vi "Arrange GU Dialog.vi"(6 "Enabled Site":i32[](array[numeric])=[0, 2], 7 "CAL Config File Path":path=path "C:/Users/Public/Documents/National Instruments/Golden Units Calibration Tool/Calibration Config/Golden Units Calibration.csv", 8 "error in":errorcluster, 9 "Cur Cal Type":T2=enum."Check", 10 "All Available GU":i32[](array[numeric])=[1, 2, 3], 11 "Config File Data":T1(array[cluster])=[{"Section Name"="General", "Section Data"=[["Match_SeqFile", "Golden Units Calibration.seq"], ["CorrOffsetFilePath", "C:\\Users\\Public\\Documents\\National Instruments\\TestStand 2019 (64-bit)\\Examples\\Golden Units Calibration Tool\\Supporting Materials\\Golden Units\\Offset.txt"]]}, {"Section Name"="PluginCfg", "Section Data"=[["GUCalibration.lvlib", "Enabled:TRUE;Trigger:TRUE;Option:TRUE;Limit:TRUE;Offset:TRUE;Report:TRUE"]]}, {"Section Name"="PluginSpecific", "Section Data"=[["CorrOffsetFilePath", "C:\\Users\\Public\\Documents\\National Instruments\\TestStand 2019 (64-bit)\\Examples\\Golden Units Calibration Tool\\Supporting Materials\\Golden Units\\Offset.txt"], ["GUBenchFilePath", "C:\\Users\\Public\\Documents\\National Instruments\\TestStand 2019 (64-bit)\\Examples\\Golden Units Calibration Tool\\Supporting Materials\\Golden Units\\GU_Bench.csv"], ["IsCalibration", "FALSE"]]}, {"Section Name"="CalCfg", "Section Data"=[["Index", "TestName", "TestNumber", "Units", "LowLimit", "HighLimit", "GU_1"], ["1", "TXP - Average Mean Power", "1001", "dBm", "-13", "-11", "0"], ["2", "TXP - Peak to Average Ratio", "1002", "dB", "9", "11", "0"], ["3", "TXP - Maximum Power", "1003", "dBm", "-3", "-1", "0"], ["4", "TXP - Minimum Power", "1004", "dBm", "0", "0", "0"], ["5", "AMPM - Mean RMS EVM", "2001", "%", "0.1", "0.3", "0"], ["6", "AMPM - Mean Linear Gain", "2002", "dB", "-4", "-2", "0"]]}]) -> (0 "error out":errorcluster, 1 "Msg":string, 3 "Config File.Data":T1(array[cluster])=[{"Section Name"="General", "Section Data"=[["Match_SeqFile", "Golden Units Calibration.seq"], ["CorrOffsetFilePath", "C:\\Users\\Public\\Documents\\National Instruments\\TestStand 2019 (64-bit)\\Examples\\Golden Units Calibration Tool\\Supporting Materials\\Golden Units\\Offset.txt"]]}, {"Section Name"="PluginCfg", "Section Data"=[["GUCalibration.lvlib", "Enabled:TRUE;Trigger:TRUE;Option:TRUE;Limit:TRUE;Offset:TRUE;Report:TRUE"]]}, {"Section Name"="PluginSpecific", "Section Data"=[["CorrOffsetFilePath", "C:\\Users\\Public\\Documents\\National Instruments\\TestStand 2019 (64-bit)\\Examples\\Golden Units Calibration Tool\\Supporting Materials\\Golden Units\\Offset.txt"], ["GUBenchFilePath", "C:\\Users\\Public\\Documents\\National Instruments\\TestStand 2019 (64-bit)\\Examples\\Golden Units Calibration Tool\\Supporting Materials\\Golden Units\\GU_Bench.csv"], ["IsCalibration", "FALSE"]]}, {"Section Name"="CalCfg", "Section Data"=[["Index", "TestName", "TestNumber", "Units", "LowLimit", "HighLimit", "GU_1"], ["1", "TXP - Average Mean Power", "1001", "dBm", "-13", "-11", "0"], ["2", "TXP - Peak to Average Ratio", "1002", "dB", "9", "11", "0"], ["3", "TXP - Maximum Power", "1003", "dBm", "-3", "-1", "0"], ["4", "TXP - Minimum Power", "1004", "dBm", "0", "0", "0"], ["5", "AMPM - Mean RMS EVM", "2001", "%", "0.1", "0.3", "0"], ["6", "AMPM - Mean Linear Gain", "2002", "dB", "-4", "-2", "0"]]}, {"Section Name"="Backup", "Section Data"=[["CorrOffsetFilePath", "C:\\Users\\Public\\Documents\\National Instruments\\TestStand 2019 (64-bit)\\Examples\\Golden Units Calibration Tool\\Supporting Materials\\Golden Units\\Offset.txt"], ["GUBenchFilePath", "C:\\Users\\Public\\Documents\\National Instruments\\TestStand 2019 (64-bit)\\Examples\\Golden Units Calibration Tool\\Supporting Materials\\Golden Units\\GU_Bench.csv"], ["IsCalibration", "FALSE"]]}])   [LabVIEW 2020, in "GUCalibration2.lvlib"]
uses:
  GUCalibration2.lvlib
  Controls/CalibrationOrCheck.ctl
  Controls/GU Arrange UI Ref.ctl
  Controls/Config Data Type.ctl
  Controls/GU Arrange Check Rule.ctl
panel:
  in  "Tab":enum32{"GU Selection", "GU Distribution"}(tab)
  in  "Abort":bool
  in  "Next":bool
  out "Selected GU List":i32(listbox)
  in  "Availabe GU List":i32(listbox)
  in  "Select All":bool
  in  "Select None":bool
  in  "GU Arrange List":i32(listbox)
  in  "Auto Arrange":bool
  in  "OK":bool
  in  "Back":bool
  in  "Loop Count per GU":i32=1 min=1 step=1
  in  "Min Num of Pass GUs per Site":i32=1 min=1 step=1
  # "Select GUs"
  # "GU Arrangements"
  # "Arrangement"
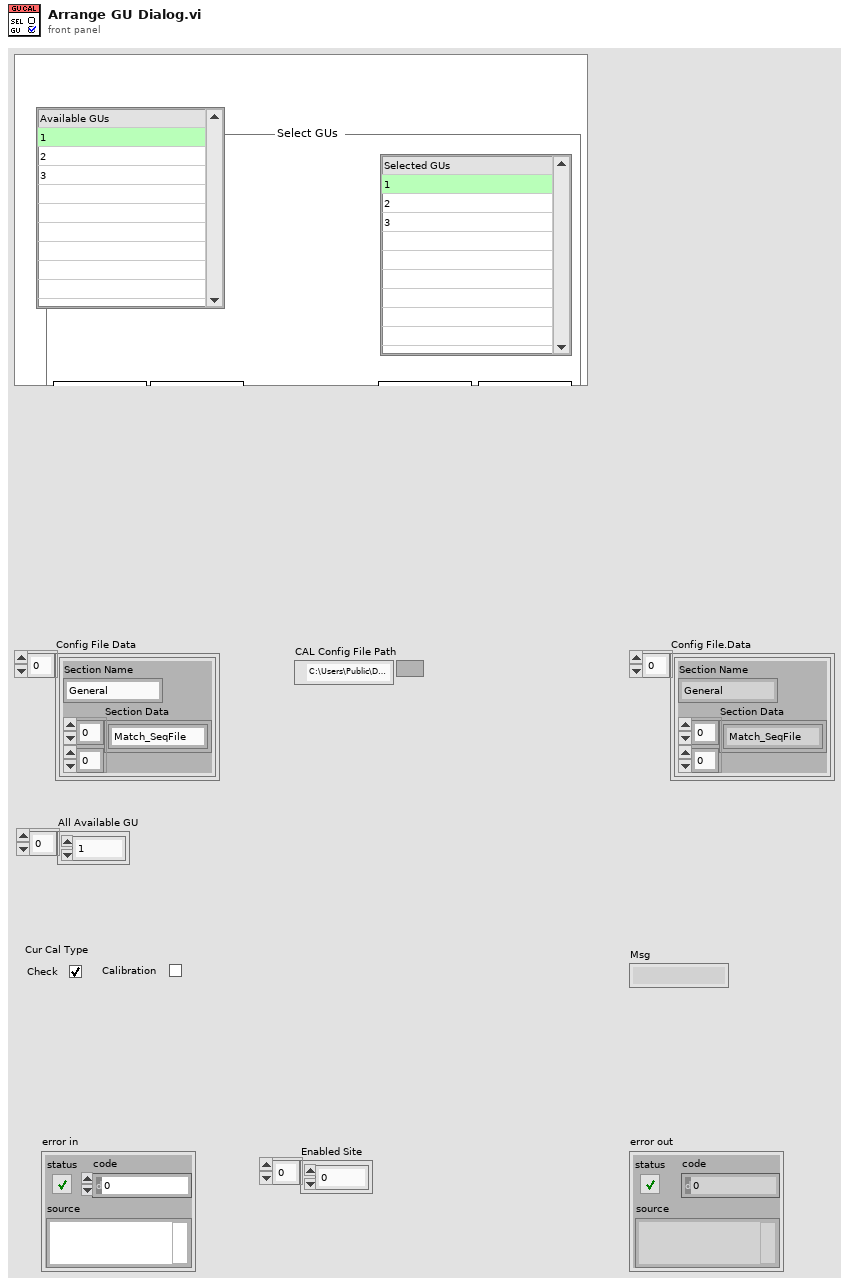
[diagram p1: front panel]
types:
  T1 = cluster{"Section Name":string, "Section Data":string[][]}[]
  T2 = typedef "GUCalibration2.lvlib/CalibrationOrCheck.ctl" = enum32{"Calibration", "Check"}
  T3 = typedef "GUCalibration2.lvlib/GU Arrange UI Ref.ctl" = cluster{"Availabe GU List":refnum<vi>, "Selected GU List":refnum<vi>, "Tab":refnum<vi>, "GU Arrange List":refnum<vi>, "Loop Count Per Batch":refnum<vi>, "This VI":refnum<vi>, "Min Num of Pass Batch":refnum<vi>}
  T4 = typedef "GUCalibration2.lvlib/Config Data Type.ctl" = cluster{"Cal Type":i32, "Curr Batch Index":i32, "Loop Count Per GU":i32, "Min Num of Pass GUs Per Site":i32, "Is Calibration":bool, "Batch Iteration Done":bool, "Cal Abort":bool, "Update Offset":bool, "Cal Check Pass":bool, "Cal End":bool, "Enabled Site":i32[], "GU Selected":i32[], "All Available GU":i32[], "GU Arrange":i32[][], "Batch Test Count":i32[][], "Batch Test Result":string[][], "Curr Batch":i32[], "Curr Batch Test Count":i32[], "Curr Batch Target Count":i32[], "Curr Batch Test Result":string[]}
  T5 = typedef "GUCalibration2.lvlib/GU Arrange Check Rule.ctl" = enum16{"Invalid GU Number", "GU Number Conflict"}
  T6 = cluster{"Error In":errorcluster, "Config File":cluster{"Path":path, "Data":cluster{"Section Name":string, "Section Data":string[][]}[], "Data Backup":cluster{"Section Name":string, "Section Data":string[][]}[]}, "Ctrl Ref":T3, "Latest Cal Data":T4, "Curr Cal Cfg":T4, "Items Pre Edit":string[][], "Error Cell":cluster{"Cell Pos":cluster{"Row":i32, "Column":i32}[], "Error Msg":T5}[], "Exit":bool, "msg":string}
  T7 = typedef "LVPoint32TypeDef.ctl" = cluster{"Horizontal":i32, "Vertical":i32}
  T8 = typedef "LVRowAndColumnTypeDef.ctl" = cluster{"Row":i32, "Column":i32}
  T9 = cluster{"Cell Pos":cluster{"Row":i32, "Column":i32}[], "Error Msg":T5}[]
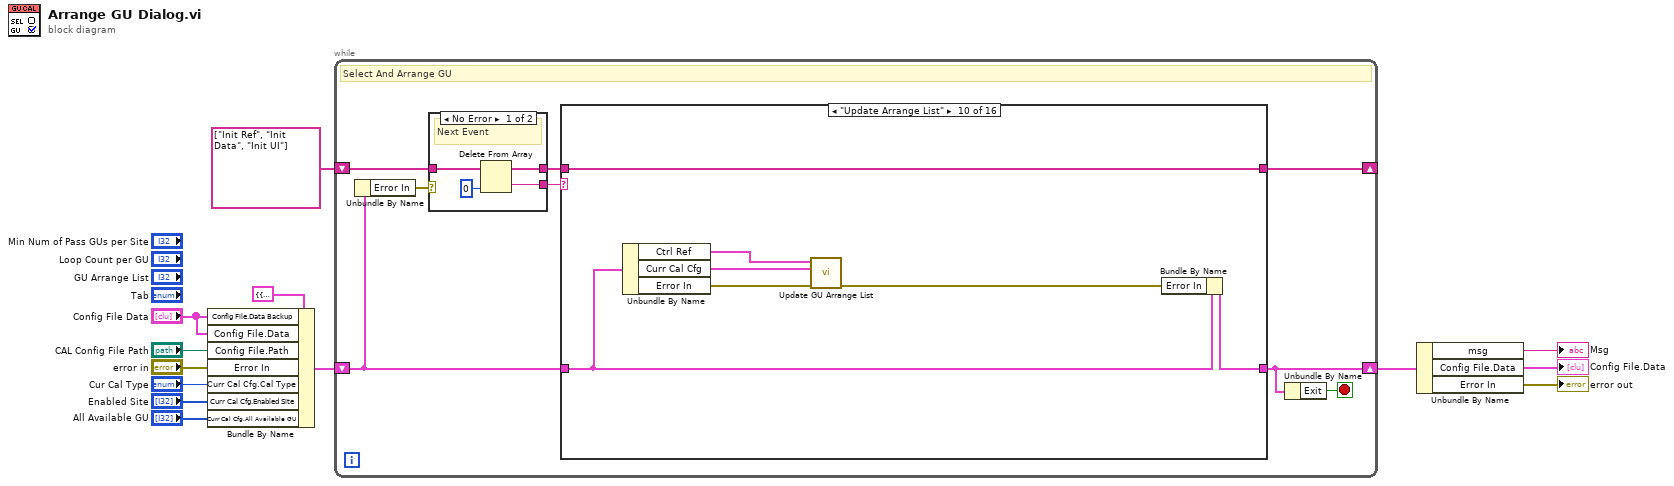
[diagram p0: block diagram]
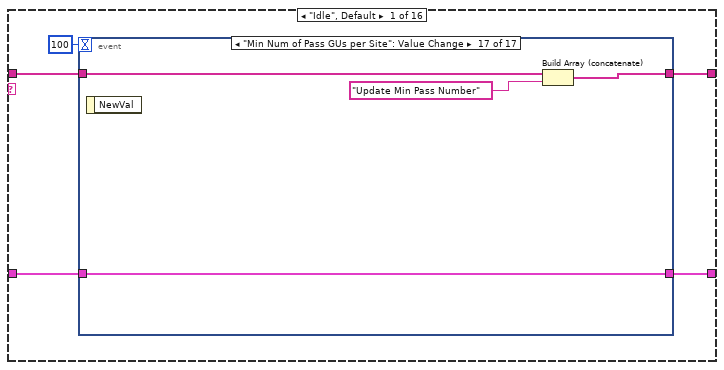
[diagram p2: hidden frame]
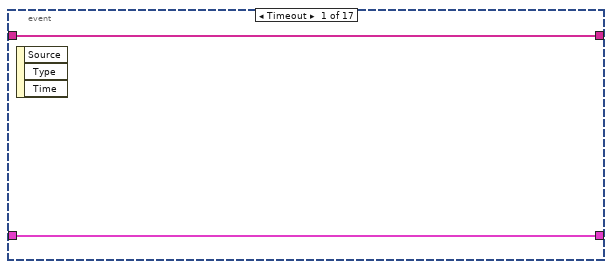
[diagram p3: hidden frame]
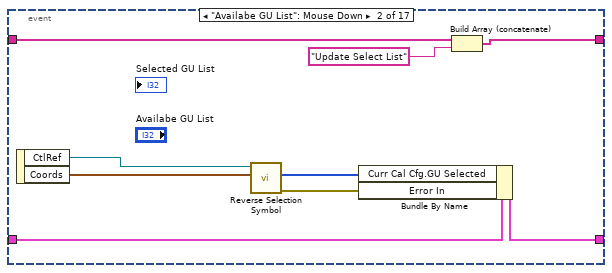
[diagram p4: hidden frame]
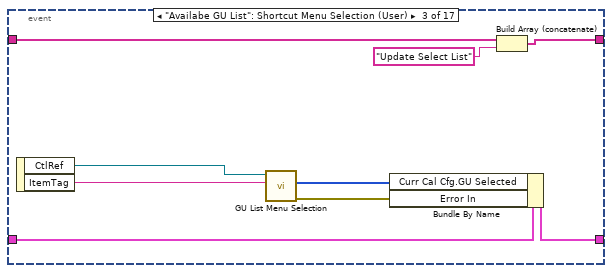
[diagram p5: hidden frame]
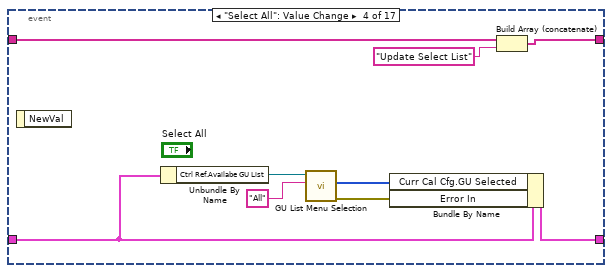
[diagram p6: hidden frame]
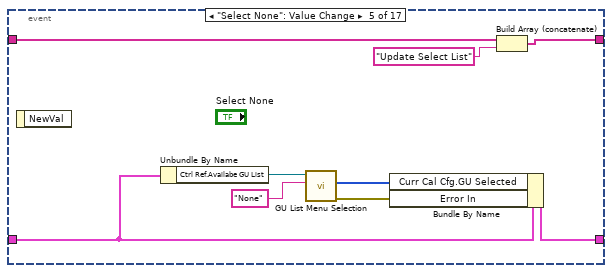
[diagram p7: hidden frame]
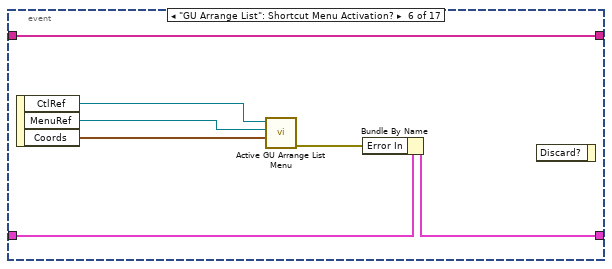
[diagram p8: hidden frame]
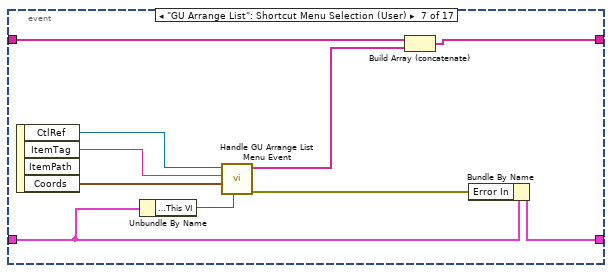
[diagram p9: hidden frame]
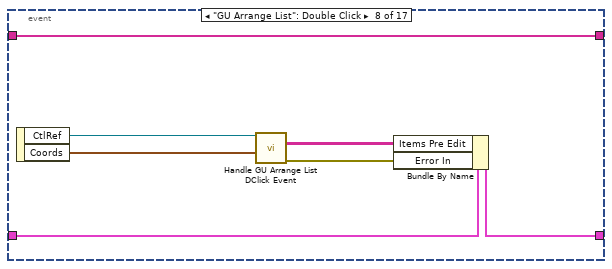
[diagram p10: hidden frame]
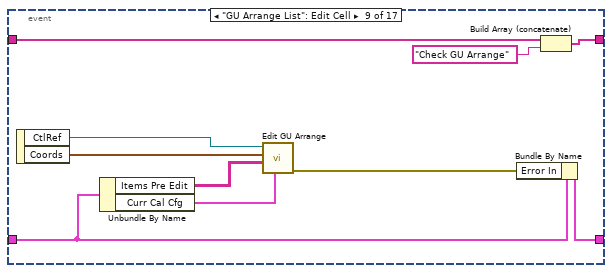
[diagram p11: hidden frame]
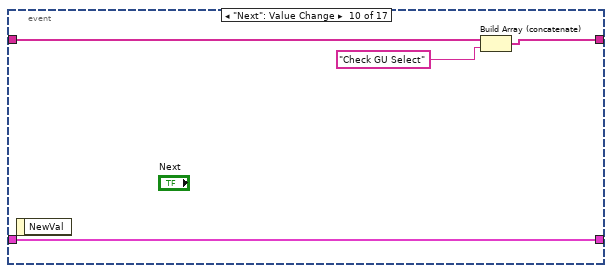
[diagram p12: hidden frame]
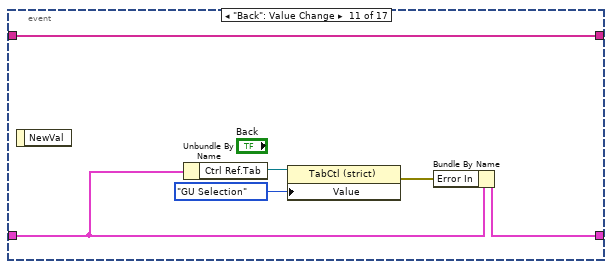
[diagram p13: hidden frame]
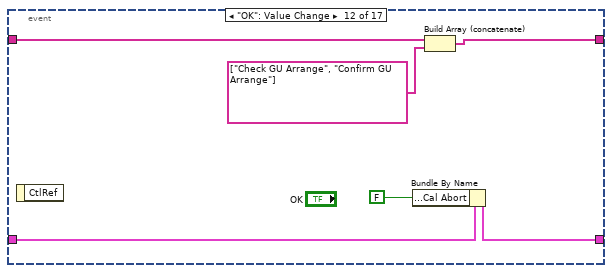
[diagram p14: hidden frame]
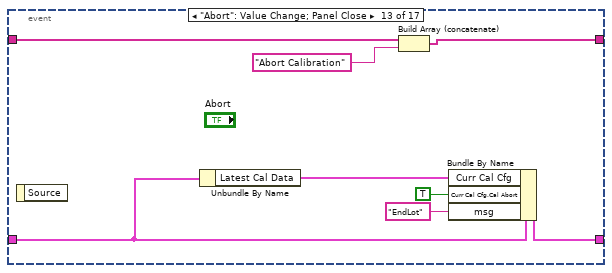
[diagram p15: hidden frame]
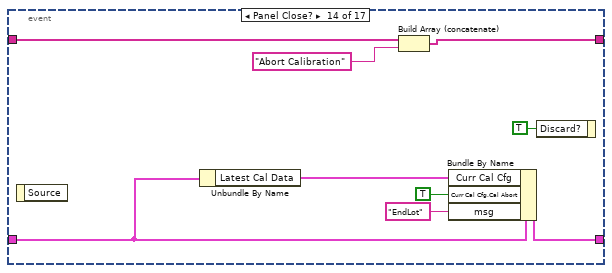
[diagram p16: hidden frame]
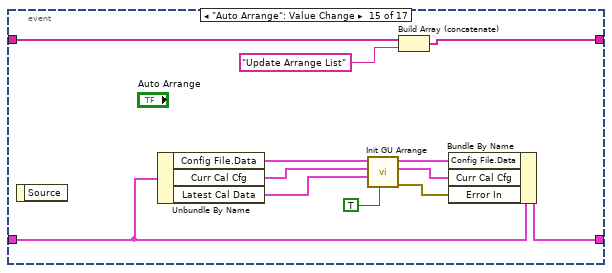
[diagram p17: hidden frame]
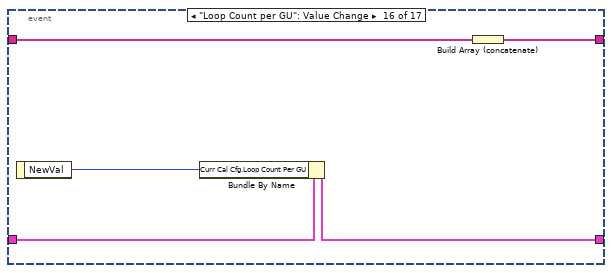
[diagram p18: hidden frame]
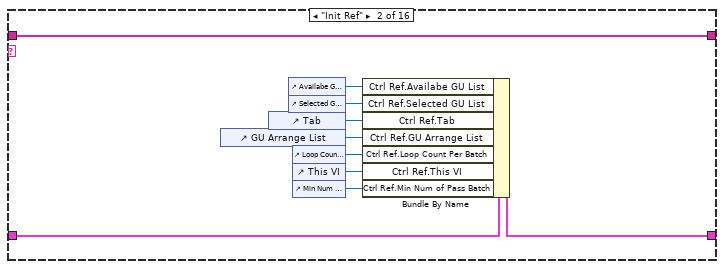
[diagram p19: hidden frame]
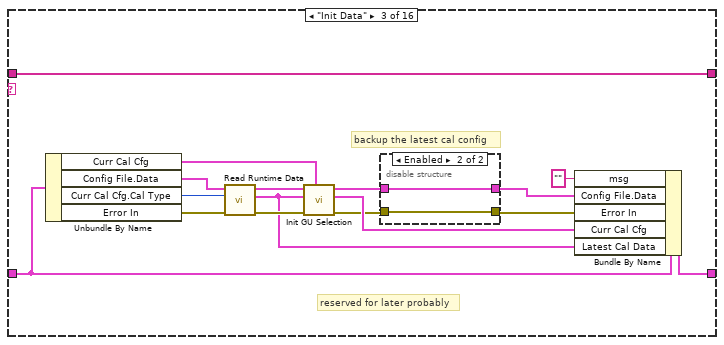
[diagram p20: hidden frame]
diagram:
  n1 = Bundle By Name(cluster=T6 {"Error In"={"status"=FALSE, "code"=0, "source"=""}, "Config File"={"Path"=path "", "Data"=[], "Data Backup"=[]}, "Ctrl Ref"={"Availabe GU List"=refnum, "Selected GU List"=refnum, "Tab"=refnum, "GU Arrange List"=refnum, "Loop Count Per Batch"=refnum, "This VI"=refnum, "Min Num of Pass Batch"=refnum}, "Latest Cal Data"={"Cal Type"=0, "Curr Batch Index"=0, "Loop Count Per GU"=0, "Min Num of Pass GUs Per Site"=0, "Is Calibration"=FALSE, "Batch Iteration Done"=FALSE, "Cal Abort"=FALSE, "Update Offset"=FALSE, "Cal Check Pass"=FALSE, "Cal End"=FALSE, "Enabled Site"=[], "GU Selected"=[], "All Available GU"=[], "GU Arrange"=[], "Batch Test Count"=[], "Batch Test Result"=[], "Curr Batch"=[], "Curr Batch Test Count"=[], "Curr Batch Target Count"=[], "Curr Batch Test Result"=[]}, "Curr Cal Cfg"={"Cal Type"=0, "Curr Batch Index"=0, "Loop Count Per GU"=0, "Min Num of Pass GUs Per Site"=0, "Is Calibration"=FALSE, "Batch Iteration Done"=FALSE, "Cal Abort"=FALSE, "Update Offset"=FALSE, "Cal Check Pass"=FALSE, "Cal End"=FALSE, "Enabled Site"=[], "GU Selected"=[], "All Available GU"=[], "GU Arrange"=[], "Batch Test Count"=[], "Batch Test Result"=[], "Curr Batch"=[], "Curr Batch Test Count"=[], "Curr Batch Target Count"=[], "Curr Batch Test Result"=[]}, "Items Pre Edit"=[], "Error Cell"=[], "Exit"=FALSE, "msg"=""} ("Temp Var"), "Config File.Data Backup"="Config File Data", "Config File.Data"="Config File Data", "Config File.Path"="CAL Config File Path", "Error In"="error in", "Curr Cal Cfg.Cal Type"="Cur Cal Type", "Curr Cal Cfg.Enabled Site"="Enabled Site", "Curr Cal Cfg.All Available GU"="All Available GU") -> (w10:T6)
  n2 = while {
    shift-right: [w18] -> _
    shift-left: string[] ["Init Ref", "Init Data", "Init UI"] ("Array") -> [w21]
    shift-right: [w15] -> w9
    shift-left: w10 -> [w14]
    stop <- w16 stop-if-true
    # "Select And Arrange GU"
    n3 = Unbundle By Name(w14) -> ("Error In"=w20:errorcluster)
    n4 = case shown="No Error" w20 {
      tunnel: w21 -> [w310 w312]
      tunnel: [w308 w312] -> w19
      tunnel: [w307 "Error Handle" ("String")] -> w17
      frame No Error {
        # "Next Event"
        n5 = Delete From Array(array=w310, index=0) -> (deleted portion=w307:string, array with subset deleted=w308:string[])  [unwired: 1 in]
      }
      frame Error {
        # "Error Event"
      }
    }
    n6 = case shown="\"Update Arrange List\"" w17 {
      tunnel: [w25 w160 w176 w195 w203 w208 w213 w217 w218 w229 w240 w253 w265 w279 w295 w299] -> w15
      tunnel: w14 -> [w24 w161 w175 w194 w204 w209 w214 w217 w219 w230 w242 w251 w266 w280 w296 w300]
      tunnel: w19 -> [w23 w162 w178 w196 w205 w211 w215 w216 w224 w231 w243 w254 w272 w275 w293 w306]
      tunnel: [w22 w162 w178 w196 w205 w211 w215 w216 w224 w231 w243 w245 w263 w274 w292 w306] -> w18
      frame "Idle", Default {
        n7 = event shown="[16] \"Min Num of Pass GUs per Site\": Value Change" {
          selector: _ -> [_ _ _ _ _ _ _ _ _ _ _ _ _ _ _ _ _]
          dyn-events: _ -> [_ _ _ _ _ _ _ _ _ _ _ _ _ _ _ _ _]
          timeout: 100 -> [_ _ _ _ _ _ _ _ _ _ _ _ _ _ _ _ _]
          tunnel: [w28 w33 w43 w55 w64 w66 w78 w86 w93 w101 w104 w111 w122 w131 w143 w146 w149] -> w25
          tunnel: w24 -> [w28 w34 w46 w49 w58 w71 w73 w88 w98 w101 w107 w109 w117 w126 w140 w148 w149]
          tunnel: w23 -> [w27 w37 w39 w51 w60 w70 w76 w87 w91 w102 w108 w114 w119 w128 w142 w147 w152]
          tunnel: [w27 w30 w38 w50 w59 w70 w74 w87 w90 w100 w108 w113 w118 w127 w141 w144 w151] -> w22
          event Timeout {
            n8 = event-data() -> ()  [unwired: 1 in, 3 out]
          }
          event "Availabe GU List": Mouse Down {
            n9 = event-data() -> ("CtlRef"=w35:refnum<vi>, "Coords"=w36:T7)  [unwired: 1 in]
            n10 = call "Reverse Selection Symbol.vi"("Coords"=w36, "GU List Ref"=w35) -> ("error out"=w32:errorcluster, "Selected GU"=w31:i32[])  [unwired: 8 in]
            n11 = Bundle By Name(cluster=w34, "Curr Cal Cfg.GU Selected"=w31, "Error In"=w32) -> (w33:T6)
            n12 = Build Array (concatenate)(w37, "Update Select List" ("String")) -> (w30:string[])
          }
          event "Availabe GU List": Shortcut Menu Selection (User) {
            n13 = event-data() -> ("CtlRef"=w45:refnum<vi>, "ItemTag"=w44:string)  [unwired: 1 in]
            n14 = call "GU List Menu Selection.vi"("ItemTag"=w44, "CtlRef"=w45) -> ("error out"=w42:errorcluster, "Selected GU"=w41:i32[])  [unwired: 8 in]
            n15 = Bundle By Name(cluster=w46, "Curr Cal Cfg.GU Selected"=w41, "Error In"=w42) -> (w43:T6)
            n16 = Build Array (concatenate)(w39, "Update Select List" ("String")) -> (w38:string[])
          }
          event "Select All": Value Change {
            n17 = event-data() -> ()  [unwired: 1 in, 1 out]
            n18 = Unbundle By Name(w49) -> ("Ctrl Ref.Availabe GU List"=w48:refnum<vi>)
            n19 = call "GU List Menu Selection.vi"("ItemTag"="All", "CtlRef"=w48) -> ("error out"=w54:errorcluster, "Selected GU"=w53:i32[])  [unwired: 8 in]
            n20 = Bundle By Name(cluster=w49, "Curr Cal Cfg.GU Selected"=w53, "Error In"=w54) -> (w55:T6)
            n21 = Build Array (concatenate)(w51, "Update Select List" ("String")) -> (w50:string[])
          }
          event "Select None": Value Change {
            n22 = event-data() -> ()  [unwired: 1 in, 1 out]
            n23 = Unbundle By Name(w58) -> ("Ctrl Ref.Availabe GU List"=w57:refnum<vi>)
            n24 = call "GU List Menu Selection.vi"("ItemTag"="None", "CtlRef"=w57) -> ("error out"=w63:errorcluster, "Selected GU"=w62:i32[])  [unwired: 8 in]
            n25 = Bundle By Name(cluster=w58, "Curr Cal Cfg.GU Selected"=w62, "Error In"=w63) -> (w64:T6)
            n26 = Build Array (concatenate)(w60, "Update Select List" ("String")) -> (w59:string[])
          }
          event "GU Arrange List": Shortcut Menu Activation? {
            n27 = event-data() -> ("CtlRef"=w69:refnum<vi>, "MenuRef"=w68:refnum<k9>, "Coords"=w67:T7)  [unwired: 1 in]
            n28 = call "Active GU Arrange List Menu.vi"("Point"=w67, "MenuRef"=w68, "CtlRef"=w69) -> ("error out"=w65:errorcluster)  [unwired: 8 in]
            n29 = Bundle By Name(cluster=w71, "Error In"=w65) -> (w66:T6)
            n30 = event-data() -> ()  [unwired: 2 in, 1 out]
          }
          event "GU Arrange List": Shortcut Menu Selection (User) {
            n31 = event-data() -> ("CtlRef"=w79:refnum<vi>, "ItemTag"=w80:string, "Coords"=w81:T7)  [unwired: 1 in, 1 out]
            n32 = Unbundle By Name(w73) -> ("Ctrl Ref.This VI"=w72:refnum<vi>)
            n33 = call "Handle GU Arrange List Menu Event.vi"("Top VI"=w72, "Coords"=w81, "ItemTag"=w80, "CtlRef"=w79) -> ("error out"=w77:errorcluster, "Next Case"=w75:string[])  [unwired: 6 in]
            n34 = Build Array (concatenate)(w76, w75) -> (w74:string[])
            n35 = Bundle By Name(cluster=w73, "Error In"=w77) -> (w78:T6)
          }
          event "GU Arrange List": Double Click {
            n36 = event-data() -> ("CtlRef"=w85:refnum<vi>, "Coords"=w84:T7)  [unwired: 1 in]
            n37 = call "Handle GU Arrange List DClick Event.vi"("Coords"=w84, "CtlRef"=w85) -> ("error out"=w83:errorcluster, "Item Names"=w82:string[][])  [unwired: 8 in]
            n38 = Bundle By Name(cluster=w88, "Items Pre Edit"=w82, "Error In"=w83) -> (w86:T6)
          }
          event "GU Arrange List": Edit Cell {
            n39 = event-data() -> ("CtlRef"=w95:refnum<vi>, "Coords"=w96:T8)  [unwired: 1 in]
            n40 = Unbundle By Name(w98) -> ("Items Pre Edit"=w97:string[][], "Curr Cal Cfg"=w94:T4)
            n41 = call "Edit GU Arrange.vi"("Curr Cal Cfg In"=w94, "Items Pre Edit"=w97, "Coords"=w96, "CtlRef"=w95) -> ("error out"=w92:errorcluster)  [unwired: 7 in]
            n42 = Bundle By Name(cluster=w98, "Error In"=w92) -> (w93:T6)
            n43 = Build Array (concatenate)(w91, "Check GU Arrange" ("String")) -> (w90:string[])
          }
          event "Next": Value Change {
            n44 = event-data() -> ()  [unwired: 1 in, 1 out]
            n45 = Build Array (concatenate)(w102, "Check GU Select" ("String")) -> (w100:string[])
          }
          event "Back": Value Change {
            n46 = event-data() -> ()  [unwired: 1 in, 1 out]
            n47 = Unbundle By Name(w107) -> ("Ctrl Ref.Tab"=w106:refnum<vi>)
            n48 = property class="TabCtl (strict)"(reference=w106, "Value"=enum32{"GU Selection", "GU Distribution"}."GU Selection") -> (error out=w103:errorcluster)  [unwired: 1 in, 1 out]
            n49 = Bundle By Name(cluster=w107, "Error In"=w103) -> (w104:T6)
          }
          event "OK": Value Change {
            n50 = event-data() -> ()  [unwired: 1 in, 1 out]
            n51 = Bundle By Name(cluster=w109, "Curr Cal Cfg.Cal Abort"=FALSE ("Cal Abort")) -> (w111:T6)
            n52 = Build Array (concatenate)(w114, string[] ["Check GU Arrange", "Confirm GU Arrange"] ("Array")) -> (w113:string[])
          }
          event "Abort": Value Change; Panel Close {
            n53 = event-data() -> ()  [unwired: 1 in, 1 out]
            n54 = Unbundle By Name(w117) -> ("Latest Cal Data"=w116:T4)
            n55 = Build Array (concatenate)(w119, "Abort Calibration" ("msg")) -> (w118:string[])
            n56 = Bundle By Name(cluster=w117, "Curr Cal Cfg"=w116, "Curr Cal Cfg.Cal Abort"=TRUE, "msg"="EndLot") -> (w122:T6)
          }
          event Panel Close? {
            n57 = event-data() -> ()  [unwired: 1 in, 1 out]
            n58 = Unbundle By Name(w126) -> ("Latest Cal Data"=w125:T4)
            n59 = Build Array (concatenate)(w128, "Abort Calibration" ("msg")) -> (w127:string[])
            n60 = Bundle By Name(cluster=w126, "Curr Cal Cfg"=w125, "Curr Cal Cfg.Cal Abort"=TRUE, "msg"="EndLot") -> (w131:T6)
            n61 = event-data("Discard?"=TRUE) -> ()  [unwired: 1 in, 1 out]
          }
          event "Auto Arrange": Value Change {
            n62 = event-data() -> ()  [unwired: 1 in, 1 out]
            n63 = Unbundle By Name(w140) -> ("Config File.Data"=w138:T1, "Curr Cal Cfg"=w137:T4, "Latest Cal Data"=w136:T4)
            n64 = call "Init GU Arrange.vi"("Force Auto(False)"=TRUE, "Latest Cal Cfg"=w136, "Curr Cal Cfg In"=w137, "Config Data"=w138) -> ("error out"=w133:errorcluster, "Curr Cal Cfg Out"=w134:T4, "Config Data Out"=w135:T1)  [unwired: 5 in]
            n65 = Build Array (concatenate)(w142, "Update Arrange List" ("msg")) -> (w141:string[])
            n66 = Bundle By Name(cluster=w140, "Config File.Data"=w135, "Curr Cal Cfg"=w134, "Error In"=w133) -> (w143:T6)
          }
          event "Loop Count per GU": Value Change {
            n67 = event-data() -> ("NewVal"=w145:i32)  [unwired: 1 in]
            n68 = Bundle By Name(cluster=w148, "Curr Cal Cfg.Loop Count Per GU"=w145) -> (w146:T6)
            n69 = Build Array (concatenate)(w147) -> (w144:string[])
          }
          event "Min Num of Pass GUs per Site": Value Change {
            n70 = event-data() -> ()  [unwired: 1 in, 1 out]
            n71 = Build Array (concatenate)(w152, "Update Min Pass Number" ("String")) -> (w151:string[])
          }
        }
      }
      frame "Init Ref" {
        n72 = control-ref of="GU Arrange List"() -> (w156:refnum<vi>)
        n73 = control-ref of="Tab"() -> (w157:refnum<vi>)
        n74 = control-ref of="Availabe GU List"() -> (w159:refnum<vi>)
        n75 = control-ref of="Selected GU List"() -> (w158:refnum<vi>)
        n76 = control-ref of="Loop Count per GU"() -> (w155:refnum<vi>)
        n77 = control-ref of="This VI"() -> (w154:refnum<vi>)
        n78 = control-ref of="Min Num of Pass GUs per Site"() -> (w153:refnum<vi>)
        n79 = Bundle By Name(cluster=w161, "Ctrl Ref.Availabe GU List"=w159, "Ctrl Ref.Selected GU List"=w158, "Ctrl Ref.Tab"=w157, "Ctrl Ref.GU Arrange List"=w156, "Ctrl Ref.Loop Count Per Batch"=w155, "Ctrl Ref.This VI"=w154, "Ctrl Ref.Min Num of Pass Batch"=w153) -> (w160:T6)
      }
      frame "Init Data" {
        # "reserved for later probably"
        # "backup the latest cal config"
        n80 = Unbundle By Name(w175) -> ("Curr Cal Cfg"=w168:T4, "Config File.Data"=w177:T1, "Curr Cal Cfg.Cal Type"=w163:i32, "Error In"=w167:errorcluster)
        n81 = call "Read Runtime Data.vi"("error in"=w167, "Curr Cal Type"=w163, "Config File Data In"=w177) -> ("error out"=w174:errorcluster, "Runtime Data Out"=w173:T4, "Config Data Out"=w172:T1)  [unwired: 6 in]
        n82 = call "Init GU Selection.vi"("Curr Cal Cfg In"=w168, "error in"=w174, "Latest Cal Cfg"=w173, "Config Data"=w172) -> ("error out"=w166:errorcluster, "Curr Cal Cfg Out"=w169:T4, "Config Data Out"=w165:T1)  [unwired: 5 in]
        n83 = disable-structure shown="Enabled" {
          disable-tunnel: [w184 w185] -> w171
          disable-tunnel: [w183 w186] -> w170
          disable-tunnel: w166 -> [w182 w185]
          disable-tunnel: w165 -> [w181 w186]
          frame Disabled {
            n84 = call "Remove Backup Config.vi"("error in"=w182, "Config File Data In"=w181) -> ("error out"=w179:errorcluster, "Config Data Out"=w180:T1)  [unwired: 8 in]
            n85 = call "Backup Latest Cal Config.vi"("error in"=w179, "Config File Data In"=w180) -> ("error out"=w184:errorcluster, "Config Data Out"=w183:T1)  [unwired: 8 in]
          }
          frame Enabled {
          }
        }
        n86 = Bundle By Name(cluster=w175, "msg"="", "Config File.Data"=w170, "Error In"=w171, "Curr Cal Cfg"=w169, "Latest Cal Data"=w173) -> (w176:T6)
      }
      frame "Init GU Arrange" {
        n87 = Unbundle By Name(w194) -> ("Config File.Data"=w192:T1, "Curr Cal Cfg"=w191:T4, "Latest Cal Data"=w190:T4, "Error In"=w193:errorcluster)
        n88 = call "Init GU Arrange.vi"("error in"=w193, "Latest Cal Cfg"=w190, "Curr Cal Cfg In"=w191, "Config Data"=w192) -> ("error out"=w189:errorcluster, "Curr Cal Cfg Out"=w187:T4, "Config Data Out"=w188:T1)  [unwired: 5 in]
        n89 = Bundle By Name(cluster=w194, "Config File.Data"=w188, "Curr Cal Cfg"=w187, "Error In"=w189) -> (w195:T6)
      }
      frame "Init UI" {
        n90 = Unbundle By Name(w204) -> ("Curr Cal Cfg"=w201:T4, "Ctrl Ref"=w199:T3, "Latest Cal Data.Loop Count Per GU"=w197:i32, "Error In"=w198:errorcluster)
        n91 = call "Init Front Panel Ctrls.vi"("error in"=w198, "Latest Loop Count"=w197, "Ctrl Ref"=w199) -> ("error out"=w200:errorcluster)  [unwired: 8 in]
        n92 = call "Update GU Selection List.vi"("error in"=w200, "Curr Cal Cfg"=w201, "Ctrl Ref"=w199) -> ("error out"=w202:errorcluster)  [unwired: 8 in]
        n93 = Bundle By Name(cluster=w204, "Error In"=w202) -> (w203:T6)
      }
      frame "Error Handle" {
        n94 = Unbundle By Name(w209) -> ("Error In"=w210:errorcluster)
        n95 = call <vilib>:"Simple Error Handler.vi"("error in (no error)"=w210) -> ("error out"=w207:errorcluster)  [unwired: 4 in, 4 out]
        n96 = Unbundle By Name(w207) -> ("status"=w206:bool)
        n97 = Bundle By Name(cluster=w209, "Exit"=w206, "Error In"=w207) -> (w208:T6)
      }
      frame "Exit" {
        n98 = Bundle By Name(cluster=w214, "Exit"=TRUE) -> (w213:T6)
      }
      frame "----------------" {
      }
      frame "Update Select List" {
        n99 = Unbundle By Name(w219) -> ("Ctrl Ref"=w221:T3, "Curr Cal Cfg"=w222:T4, "Error In"=w223:errorcluster)
        n100 = call "Update GU Selection List.vi"("error in"=w223, "Curr Cal Cfg"=w222, "Ctrl Ref"=w221) -> ("error out"=w220:errorcluster)  [unwired: 8 in]
        n101 = Bundle By Name(cluster=w219, "Error In"=w220) -> (w218:T6)
      }
      frame "Update Arrange List" {
        n102 = Unbundle By Name(w230) -> ("Ctrl Ref"=w226:T3, "Curr Cal Cfg"=w225:T4, "Error In"=w228:errorcluster)
        n103 = call "Update GU Arrange List.vi"("error in"=w228, "Curr Cal Cfg"=w225, "Ctrl Ref"=w226) -> ("error out"=w227:errorcluster)  [unwired: 8 in]
        n104 = Bundle By Name(cluster=w230, "Error In"=w227) -> (w229:T6)
      }
      frame "Check GU Arrange" {
        n105 = Unbundle By Name(w242) -> ("Ctrl Ref.This VI"=w232:refnum<vi>, "Ctrl Ref.GU Arrange List"=w239:refnum<vi>, "Curr Cal Cfg"=w238:T4, "Error In"=w241:errorcluster)
        n106 = call "Check GU Number Arrange.vi"("error in"=w241, "Curr Cal Cfg In"=w238, "GU Arrange List"=w239) -> ("error out"=w237:errorcluster, "Error Cell"=w236:T9, "GU Arrange List  Ref Out"=w233:refnum<vi>)  [unwired: 5 in, 1 out]
        n107 = call "Highlight the Error GU Cell.vi"("Top VI"=w232, "error in"=w237, "Error Cell"=w236, "GU Arrange List"=w233) -> ("error out"=w234:errorcluster, "Error Cell  Out"=w235:T9)  [unwired: 6 in]
        n108 = Bundle By Name(cluster=w242, "Error Cell"=w235, "Error In"=w234) -> (w240:T6)
      }
      frame "Check GU Select" {
        n109 = Unbundle By Name(w251) -> ("Ctrl Ref.Tab"=w249:refnum<vi>, "Curr Cal Cfg"=w252:T4)
        n110 = call "Check GU Selection.vi"("Curr Cal Cfg"=w252) -> ("error out"=w248:errorcluster, "Info"=w246:string, "OK?"=w250:bool)  [unwired: 7 in, 1 out]
        n111 = case shown="True" w250 {
          tunnel: w249 -> [_ w260]
          tunnel: w248 -> [w256 w259]
          tunnel: [w256 w258] -> w247
          tunnel: w246 -> [w255 _]
          tunnel: [_ string[] ["Init GU Arrange", "Update Arrange List"]] -> w244
          frame False {
            n112 = One Button Dialog(message=w255) -> ()  [unwired: 1 in, 1 out]
          }
          frame True {
            n113 = property class="TabCtl (strict)"(reference=w260, error in=w259, "Value"=enum32{"GU Selection", "GU Distribution"}."GU Distribution") -> (error out=w258:errorcluster)  [unwired: 1 out]
          }
        }
        n114 = Bundle By Name(cluster=w251, "Error In"=w247) -> (w253:T6)
        n115 = Build Array (concatenate)(w254, w244) -> (w245:string[])
      }
      frame "Confirm GU Arrange" {
        n116 = Unbundle By Name(w266) -> ("Ctrl Ref.GU Arrange List"=w271:refnum<vi>, "Curr Cal Cfg"=w270:T4, "Error Cell"=w269:T9, "Error In"=w264:errorcluster)
        n117 = call "Confirm GU Arrange Scheme.vi"("error in"=w264, "Error Cell"=w269, "Curr Cal Cfg In"=w270, "GU Arrange List"=w271) -> ("error out"=w268:errorcluster, "Curr Cal Cfg Out"=w267:T4, "Next Event"=w262:string)  [unwired: 4 in, 1 out]
        n118 = Bundle By Name(cluster=w266, "Curr Cal Cfg"=w267, "Error In"=w268) -> (w265:T6)
        n119 = Build Array (concatenate)(w272, w262) -> (w263:string[])
      }
      frame "Save Config" {
        n120 = Unbundle By Name(w280) -> ("Config File.Path"=w284:path, "Config File.Data"=w283:T1, "Curr Cal Cfg"=w276:T4)
        n121 = call "Write Runtime Data.vi"("Runtime Data In"=w276, "Config File Data In"=w283) -> ("error out"=w281:errorcluster, "Config Data Out"=w277:T1)  [unwired: 7 in, 1 out]
        n122 = call "Save CalCfg File Data.vi"("Matric Section"=string[] ["CalCfg"], "error in"=w281, "File Path"=w284, "Config Data"=w277) -> ("error out"=w282:errorcluster)  [unwired: 7 in]
        n123 = Bundle By Name(cluster=w280, "Config File.Data"=w277, "Error In"=w282) -> (w279:T6)
        n124 = Build Array (concatenate)(w275, "Exit" ("String")) -> (w274:string[])
      }
      frame "Abort Calibration" {
        n125 = Unbundle By Name(w296) -> ("Config File.Data Backup"=w287:T1, "Config File.Path"=w298:path)
        n126 = call "Write Key Boolean.vi"("Section Name"="PluginSpecific", "Key Value"=TRUE, "Key Name"="Cal_Abort" ("Section Name"), "Config Data"=w287) -> ("error out"=w286:errorcluster, "Config Data dup"=w285:T1)  [unwired: 6 in]
        n127 = call "Save CalCfg File Data.vi"("Matric Section"=string[] ["CalCfg"], "error in"=w286, "File Path"=w298, "Config Data"=w285) -> ("error out"=w297:errorcluster)  [unwired: 7 in]
        n128 = Bundle By Name(cluster=w296, "Config File.Data"=w285, "Error In"=w297) -> (w295:T6)
        n129 = Build Array (concatenate)(w293, "Exit" ("String")) -> (w292:string[])
      }
      frame "Update Min Pass Number" {
        n130 = Unbundle By Name(w300) -> ("Ctrl Ref"=w304:T3, "Curr Cal Cfg"=w303:T4, "Error In"=w305:errorcluster)
        n131 = call "Update Min Pass Number.vi"("error in"=w305, "Curr Cal Cfg"=w303, "Ctrl Ref"=w304) -> ("error out"=w302:errorcluster, "Curr Cal Cfg Out"=w301:T4)  [unwired: 7 in]
        n132 = Bundle By Name(cluster=w300, "Curr Cal Cfg"=w301, "Error In"=w302) -> (w299:T6)
      }
    }
    n133 = Unbundle By Name(w15) -> ("Exit"=w16:bool)
  }
  n134 = Unbundle By Name(w9) -> ("msg"=→"Msg":string, "Config File.Data"=→"Config File.Data":T1, "Error In"=→"error out":errorcluster)
